vi "Shooter.vi"(7 "Action":T1=enum."Shoot", 8 "error in":errorcluster) -> (0 "error out":errorcluster)   [LabVIEW 2013]
doc: "Shooter is used to interact ONLY with the shooter pneumatics (kicker and firing cylinder). It can be used on its own or inside CheckedShooter.vi. It has the following actions:\n-Init: takes a single solenoid reference for the kicker and firing cylinder and passes them onto the single solenoid VI.\n-Shoot:\n +Actuates the firing cylinders.\n +Waits a specified amount of time (Wait1).\n +Actuates the kicker.\n +Waits a specified amount of time (Wait2).\n +Retracts the kicker.\n +Waits a specified amount of time (Wait3).\n +Retracts the firing cylinders."
uses:
  ShooterAction.ctl
  SingleSolenoidAction.ctl
panel:
  in  "Wait3":u32
  in  "Wait2":u32
  in  "Wait1":u32
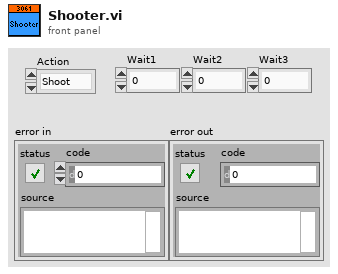
[diagram p1: front panel]
types:
  T1 = typedef "ShooterAction.ctl" = enum16{"Init", "Shoot"}
  T2 = typedef "SingleSolenoidAction.ctl" = enum16{"Init", "SetState", "Disable"}
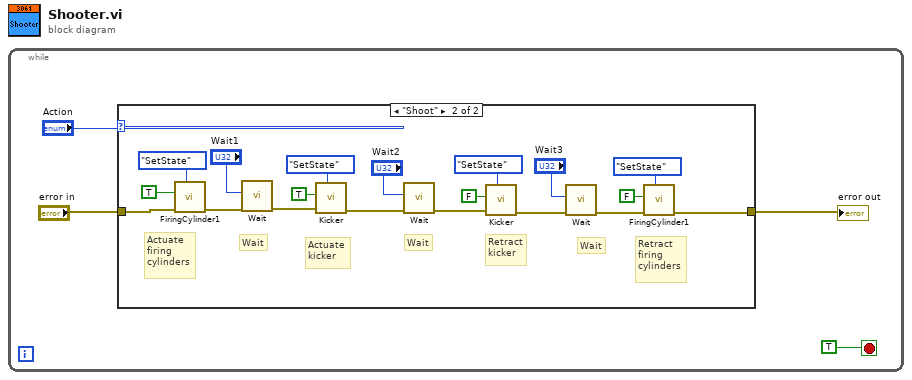
[diagram p0: block diagram]
diagram:
  n1 = while {
    stop <- TRUE stop-if-true
    n2 = case shown="\"Shoot\"" "Action" {
      tunnel: "error in" -> [w5 w16]
      tunnel: [w5 w23] -> w1
      frame "Init", Default {
        # "We shouldn't need to do anything here..."
      }
      frame "Shoot" {
        # "Retract\nfiring\ncylinders"
        # "Wait"
        # "Retract\nkicker"
        # "Wait"
        # "Actuate\nkicker"
        # "Wait"
        # "Actuate\nfiring\ncylinders"
        n3 = call "FiringCylinder1.vi"("Action"=SingleSolenoidAction."SetState" ("Mode"), "error in (no error)"=w16, "Actuate?"=TRUE ("State")) -> ("error out"=w15:errorcluster)  [unwired: 8 in]
        n4 = call "Wait.vi"("error in"=w15, "milliseconds to wait"="Wait1") -> ("error out"=w24:errorcluster)  [unwired: 9 in]
        n5 = call "Kicker.vi"("Action"=SingleSolenoidAction."SetState" ("Mode"), "error in (no error)"=w24, "Actuate?"=TRUE ("State")) -> ("error out"=w21:errorcluster)  [unwired: 8 in]
        n6 = call "Wait.vi"("error in"=w21, "milliseconds to wait"="Wait2") -> ("error out"=w20:errorcluster)  [unwired: 9 in]
        n7 = call "Kicker.vi"("Action"=SingleSolenoidAction."SetState" ("Mode"), "error in (no error)"=w20, "Actuate?"=FALSE ("State")) -> ("error out"=w19:errorcluster)  [unwired: 8 in]
        n8 = call "Wait.vi"("error in"=w19, "milliseconds to wait"="Wait3") -> ("error out"=w22:errorcluster)  [unwired: 9 in]
        n9 = call "FiringCylinder1.vi"("Action"=SingleSolenoidAction."SetState" ("Mode"), "error in (no error)"=w22, "Actuate?"=FALSE ("State")) -> ("error out"=w23:errorcluster)  [unwired: 8 in]
      }
    }
    "error out" <- w1
  }
